vi "LineFollow.vi"(3 "DC Motor":T4, 4 "Left Sensor Port":T1={"Port"=0, "MUX Port"=1} {"Port" items=["Port 1", "Port 2", "Port 3", "Port 4"]; "MUX Port" items=["No MUX", "MUX 1", "MUX 2", "MUX 3", "MUX 4"]}) -> ()   [LabVIEW 2010]
uses:
  <vilib>/NXT/HiTechnic/HiTechnic Controls/HiTechnic Port.ctl
  <vilib>/NXT/Block Support/NXT_InputPort.ctl
  <vilib>/NXT/Subs/MotorXNode.DC Motor Type.ctl
  <vilib>/NXT/Subs/LVHSConnector.ctl
  <vilib>/NXT/NXTIO Xnodes/NXTIOXNode/NXTIO.xnode
  <vilib>/NXT/Subs/MotorXNode.2DCMotor.ctl
  <vilib>/NXT/NXTIO Xnodes/NXTIONodeSubVIs/TETRIX IO Move DC Motors.vi
panel:
  in  "Right Sensor Port":T1={"Port"=0, "MUX Port"=1} {"Port" items=["Port 1", "Port 2", "Port 3", "Port 4"]; "MUX Port" items=["No MUX", "MUX 1", "MUX 2", "MUX 3", "MUX 4"]}
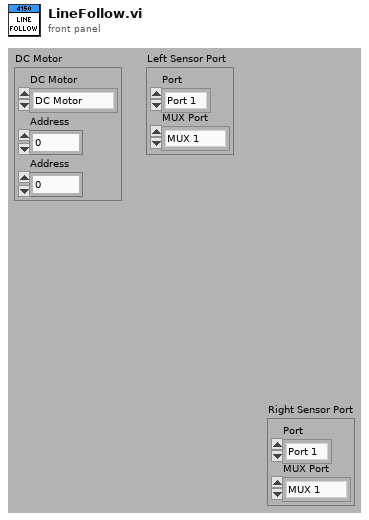
[diagram p1: front panel]
types:
  T1 = typedef "HiTechnic Port.ctl" = cluster{"Port":T2, "MUX Port":u8}
  T2 = typedef "NXT_InputPort.ctl" = u8
  T3 = typedef "MotorXNode.DC Motor Type.ctl" = enum16{"DC Motor"}
  T4 = cluster{"DC Motor":T3, "Address":i16, "Address":i16}
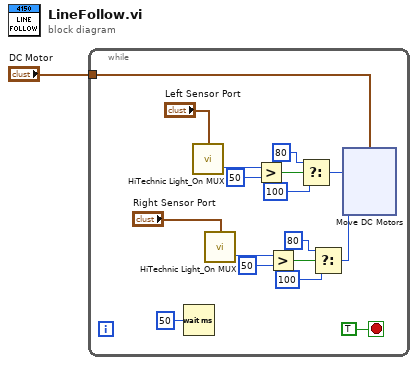
[diagram p0: block diagram]
diagram:
  n1 = while {
    tunnel: "DC Motor" -> [w17]
    stop <- TRUE stop-if-true
    n2 = Wait (ms)(milliseconds to wait=u32 50) -> ()  [unwired: 1 out]
    n3 = call <vilib>:"HiTechnic Light_On MUX.vi"("Port/MUX"="Left Sensor Port") -> ("Scaled Value"=w14:i16)  [unwired: 2 in, 1 out]
    n4 = call <vilib>:"HiTechnic Light_On MUX.vi"("Port/MUX"="Right Sensor Port") -> ("Scaled Value"=w8:i16)  [unwired: 2 in, 1 out]
    n5 = Greater?(x=w14, y=i16 50) -> (0:w12:bool)
    n6 = Greater?(x=w8, y=i16 50) -> (0:w6:bool)
    n7 = Select(t=80, s=w12, f=100) -> (s? t:f=w9:i32)
    n8 = Select(t=80, s=w6, f=100) -> (s? t:f=w2:i32)
    n9 = xnode "Move DC Motors"("Power/Speed 2"=w2, "Power/Speed 1"=w9, "Motors"=w17) -> ()  [unwired: 1 in, 1 out]
  }
